vi "OpenCloseDialogs.vi"(7 "Task":enum16{"Open", "Close"}(ring), 8 "error in (no error)":errorcluster, 11 "VI in":refnum<vi>) -> (0 "error out":errorcluster, 3 "VI out":refnum<vi>)   [LabVIEW 2022 SP3]
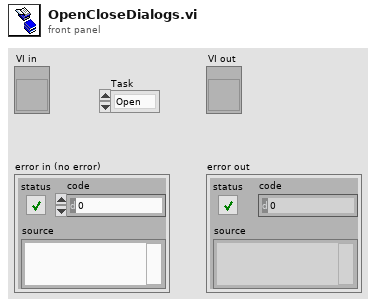
[diagram p1: front panel]
types:
  T1 = enum32{"Invalid", "Standard", "Closed", "Hidden", "Minimized", "Maximized"}
  T2 = enum32{"Invalid", "Default", "Floating", "Floating/Auto-Hide", "Modal"}
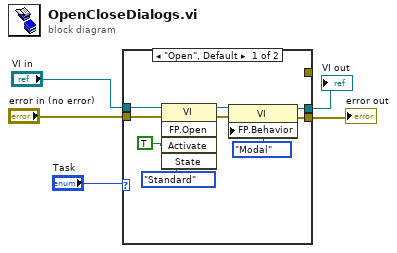
[diagram p0: block diagram]
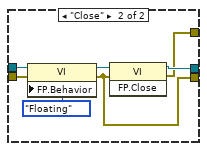
[diagram p2: hidden frame]
diagram:
  n1 = case shown="\"Open\", Default" "Task" {
    tunnel: [w14 w16] -> w5
    tunnel: [w13 w17] -> w4
    tunnel: "VI in" -> [w9 w20]
    tunnel: "error in (no error)" -> [w6 w19]
    tunnel: [_ w15] -> _
    frame "Open", Default {
      n2 = invoke class="VI" method="FP.Open"(reference=w9, error in=w6, "Activate"=TRUE ("Activate?"), "State"=T1."Standard") -> (reference out=w8:refnum<vi>, error out=w7:errorcluster)  [unwired: 1 in, 3 out]
      n3 = property class="VI"(reference=w8, error in=w7, "FP.Behavior"=T2."Modal" ("Front Panel Window:Behavior")) -> (reference out=w13:refnum<vi>, error out=w14:errorcluster)
    }
    frame "Close" {
      n4 = property class="VI"(reference=w20, error in=w19, "FP.Behavior"=T2."Floating" ("Front Panel Window:Behavior")) -> (reference out=w18:refnum<vi>, error out=w16:errorcluster)
      n5 = invoke class="VI" method="FP.Close"(reference=w18, error in=w16) -> (reference out=w17:refnum<vi>, error out=w15:errorcluster)  [unwired: 1 in, 1 out]
    }
  }
  "error out" <- w5
  "VI out" <- w4
